vi "S3Motor_control2017m.vi"() -> ()   [LabVIEW 2012]
uses:
  2015myGlobal 1.vi
panel:
  out "停留時間(秒)":dbl=4.0
  out "啟動中":u8(slide) scale=0.0..100.0
  out "#of comd":i32
  out "flag_direction":bool=TRUE
  out "Position Now":i32
  out "Set position":i32=1000
  in  "stop":bool
  out "Waveform Chart":i32(graph)
  out "Position":i32
  in  "error in (no error)":errorcluster
  out "Error Out":errorcluster={"status"=TRUE, "code"=-1073807343, "source"="VISA Write in Serial Communication for TL3T of VISA.vi"}
  in  "baud rate (9600)":u32=9600
  in  "Resource Name 0":refnum<visa-resource-name>="COM4"
  out "重複次數":i32=4
  out "速度參數":i32
  out "Step":i32
  # "Step 1: Set parameters"
  # "Step 2: Initialize Hardware"
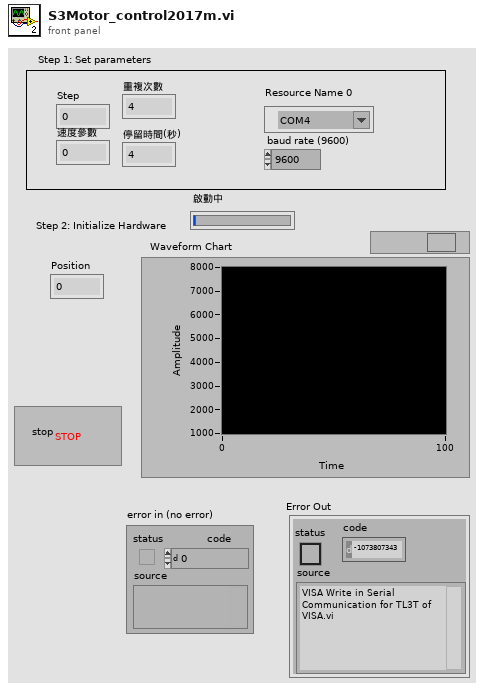
[diagram p1: front panel]
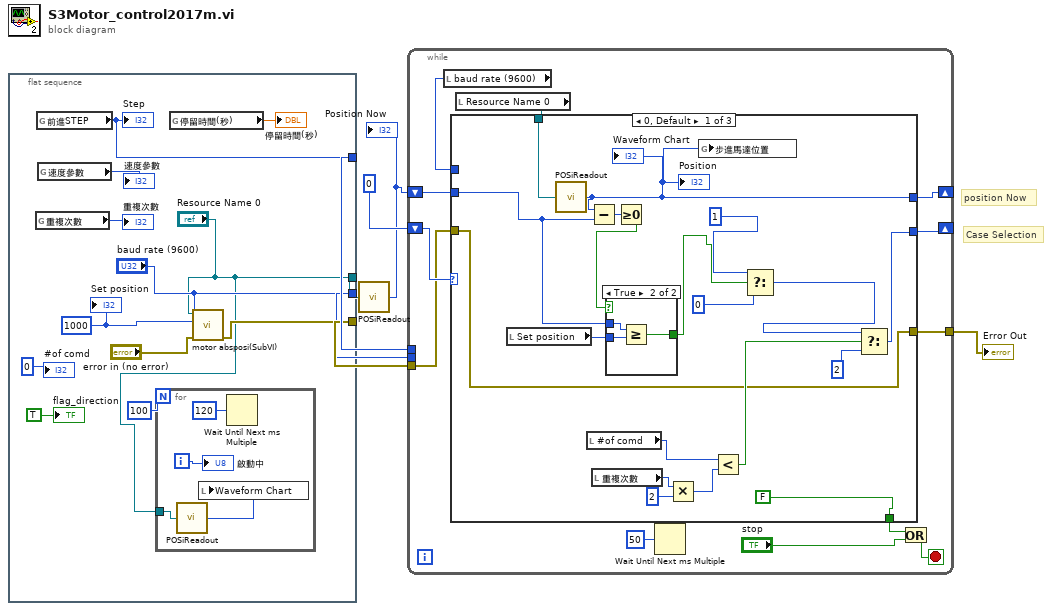
[diagram p0: block diagram]
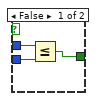
[diagram p2: hidden frame]
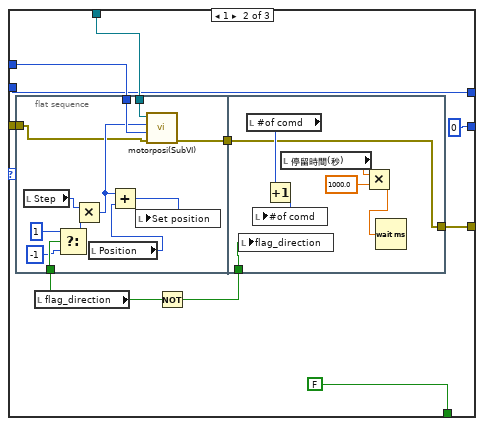
[diagram p3: hidden frame]
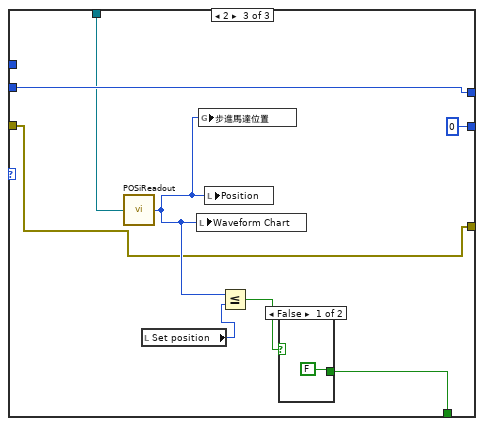
[diagram p4: hidden frame]
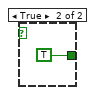
[diagram p5: hidden frame]
diagram:
  # "Case Selection"
  # "position Now"
  n1 = flat-sequence {
    tunnel: [w19] -> w7
    tunnel: ["baud rate (9600)"] -> w5
    tunnel: [w13] -> w6
    tunnel: ["Resource Name 0"] -> w3
    frame #0 {
      w16 = 1000 ("前進STEP")
      n2 = global read "2015myGlobal 1.vi" "重複次數"() -> (→"重複次數":i32)
      n3 = global read "2015myGlobal 1.vi" "前進STEP"() -> (w19:i32)
      "Step" <- w19
      n4 = global read "2015myGlobal 1.vi" "速度參數"() -> (→"速度參數":i32)
      n5 = for {
        N: 100 -> [_]
        tunnel: "Resource Name 0" -> [w21]
        i -> [w22]
        n6 = call "POSiReadout.vi"("Resource Name 0"=w21) -> ("Position number"=w20:i32)
        n7 = local write "Waveform Chart"(w20) -> ()
        n8 = Wait Until Next ms Multiple(millisecond multiple=u32 120) -> ()  [unwired: 1 out]
        "啟動中" <- w22
      }
      n9 = global read "2015myGlobal 1.vi" "停留時間(秒)"() -> (→"停留時間(秒)":dbl)
      n10 = call "motor absposi(SubVI).vi"("error in (no error)"="error in (no error)", "baud rate (9600)"="baud rate (9600)", "前進STEP"=w16, "VISA Refnum in"="Resource Name 0") -> ("error out"=w13:errorcluster)  [unwired: 6 in, 1 out]
      "Set position" <- w16
      "flag_direction" <- TRUE
      "#of comd" <- 0 ("前進STEP")
    }
  }
  n11 = call "POSiReadout.vi"("Resource Name 0"=w3) -> ("Position number"=w2:i32)
  "Position Now" <- w2
  n12 = while {
    tunnel: w7 -> [_]
    tunnel: w6 -> [w25]
    tunnel: w5 -> [_]
    shift-right: [w31] -> _
    shift-left: 0 -> [w34]
    shift-right: [w29] -> _
    shift-left: w2 -> [w30]
    tunnel: [w24] -> w1
    stop <- w26 stop-if-true
    n13 = local read "baud rate (9600)"() -> (w32:u32)
    n14 = local read "Resource Name 0"() -> (w33:refnum<visa-resource-name>)
    n15 = case shown="0, Default" w34 {
      tunnel: w33 -> [w54 w70 w94]
      tunnel: w32 -> [_ w69 _]
      tunnel: [w46 0 ("f") 0 ("f")] -> w31
      tunnel: w30 -> [w40 w67 w96]
      tunnel: [w43 w67 w96] -> w29
      tunnel: [FALSE ("stop") FALSE ("stop") w97] -> w27
      tunnel: w25 -> [w36 w63 w90]
      tunnel: [w36 w62 w90] -> w24
      frame 0, Default {
        n16 = local read "Set position"() -> (w39:i32)
        n17 = call "POSiReadout.vi"("Resource Name 0"=w54) -> ("Position number"=w43:i32)
        "Position" <- w43
        "Waveform Chart" <- w43
        n18 = local read "#of comd"() -> (w38:i32)
        n19 = Subtract(x=w43, y=w40) -> (x-y=w42:i32)
        n20 = local read "重複次數"() -> (w50:i32)
        n21 = Greater Or Equal To 0?(x=w42) -> (x >= 0?=w41:bool)
        n22 = case shown="True" w41 {
          tunnel: [w57 w60] -> w44
          tunnel: w40 -> [w56 w59]
          tunnel: w39 -> [w55 w58]
          frame False {
            n23 = Less Or Equal?(x=w56, y=w55) -> (x <= y?=w57:bool)
          }
          frame True {
            n24 = Greater Or Equal?(x=w59, y=w58) -> (x >= y?=w60:bool)
          }
        }
        n25 = Multiply(x=w50, y=2) -> (x*y=w37:i32)
        n26 = global write "2015myGlobal 1.vi" "步進馬達位置"(w43) -> ()
        n27 = Less?(x=w38, y=w37) -> (x < y?=w48:bool)
        n28 = Select(t=1, s=w44, f=0) -> (s? t:f=w47:i32)
        n29 = Select(t=w47, s=w48, f=2) -> (s? t:f=w46:i32)
      }
      frame 1 {
        n30 = flat-sequence {
          tunnel: w70 -> [w82]
          tunnel: w69 -> [w81]
          tunnel: w66 -> [w80]
          tunnel: w63 -> [w72]
          tunnel: [w71] -> w61
          tunnel: w64 -> [w89]
          tunnel: [w86] -> w62
          tunnel: w61 -> [w86]
          frame #0 {
            n31 = local read "Step"() -> (w76:i32)
            n32 = Select(t=1, s=w80, f=-1 ("t")) -> (s? t:f=w77:i32)
            n33 = Multiply(x=w76, y=w77) -> (x*y=w74:i32)
            n34 = local read "Position"() -> (w75:i32)
            n35 = Add(x=w74, y=w75) -> (x+y=w73:i32)
            n36 = local write "Set position"(w73) -> ()
            n37 = call "motorposi(SubVI).vi"("error in (no error)"=w72, "baud rate (9600)"=w81, "前進STEP"=w74, "VISA Refnum in"=w82) -> ("error out"=w71:errorcluster)  [unwired: 6 in, 1 out]
          }
          frame #1 {
            n38 = local write "flag_direction"(w89) -> ()
            n39 = local read "#of comd"() -> (w87:i32)
            n40 = Increment(x=w87) -> (x+1=w88:i32)
            n41 = local write "#of comd"(w88) -> ()
            n42 = local read "停留時間(秒)"() -> (w84:dbl)
            n43 = Multiply(x=w84, y=1000.0) -> (x*y=w83:dbl)
            n44 = Wait (ms)(milliseconds to wait=w83) -> ()  [unwired: 1 out]
          }
        }
        n45 = local read "flag_direction"() -> (w66:bool)
        n46 = Not(x=w66) -> (.not. x?=w64:bool)
      }
      frame 2 {
        n47 = call "POSiReadout.vi"("Resource Name 0"=w94) -> ("Position number"=w91:i32)
        n48 = local read "Set position"() -> (w93:i32)
        n49 = local write "Waveform Chart"(w91) -> ()
        n50 = global write "2015myGlobal 1.vi" "步進馬達位置"(w91) -> ()
        n51 = local write "Position"(w91) -> ()
        n52 = Less Or Equal?(x=w91, y=w93) -> (x <= y?=w92:bool)
        n53 = case shown="False" w92 {
          tunnel: [FALSE ("stop") TRUE ("stop")] -> w97
          frame False {
          }
          frame True {
          }
        }
      }
    }
    n54 = Wait Until Next ms Multiple(millisecond multiple=u32 50) -> ()  [unwired: 1 out]
    n55 = Or(x=w27, y="stop") -> (x .or. y?=w26:bool)
  }
  "Error Out" <- w1
